vi "Plot Load maker V2.vi"(8 "error in (no error)":errorcluster, 11 "Refs":T6) -> (0 "error out":errorcluster, 3 "Plot config":T1={"plots"=[], "X-axis"={"Name Label.Text"="", "Style"=0, "Tick Colors:Minor Tick Color"=0, "Tick Colors:Tick Color"=0, "Marker Colors:Text Color"=0, "Grid Colors:Major Color"=0, "Grid Colors:Minor Color"=0, "Mapping Mode"=0, "Flipped"=FALSE, "Name Label.Visible"=FALSE, "Name Label.Text Colors:Text Color"=0, "Scale Fit"=0, "Range:Maximum"=0.0, "Range:Minimum"=0.0, "Offset and Multiplier:Multiplier"=0.0, "Offset and Multiplier:Offset"=0.0, "Name Label.Font:Size"=0, "Marker.Font:Size"=0, "Uniform Marker Spacing?"=TRUE, "Format String"=""}, "Y-axes"=[], "General"={"Title"="", "Time to Plot"=1800.0, "Title.Visible"=FALSE, "Sidebar.Visible"=FALSE, "Plot Area:Colors:BG Color"=0, "X Scale.Plot Name"="", "X Scale.Use Plot Name"=FALSE}} {"General"."Time to Plot" format="%<%M:%S>t"})   [LabVIEW 2021, in "RocketPlot.lvlib"]
uses:
  RocketPlot.lvlib
  TypeDefs/Plot UI references.ctl
  Classes/RocketPlotHandle/RocketPlotHandle.lvclass
  <userlib>/bjustice/TipStripOOPanel/Classes/TipPanelHandle/TipPanelHandle.lvclass
  TypeDefs/Plot top row.ctl
  TypeDefs/plot load data V2.ctl
  TypeDefs/plot properties V2.ctl
  TypeDefs/plot attributes V2.ctl
  TypeDefs/Plot scale axis properties.ctl
  TypeDefs/Plot general properties.ctl
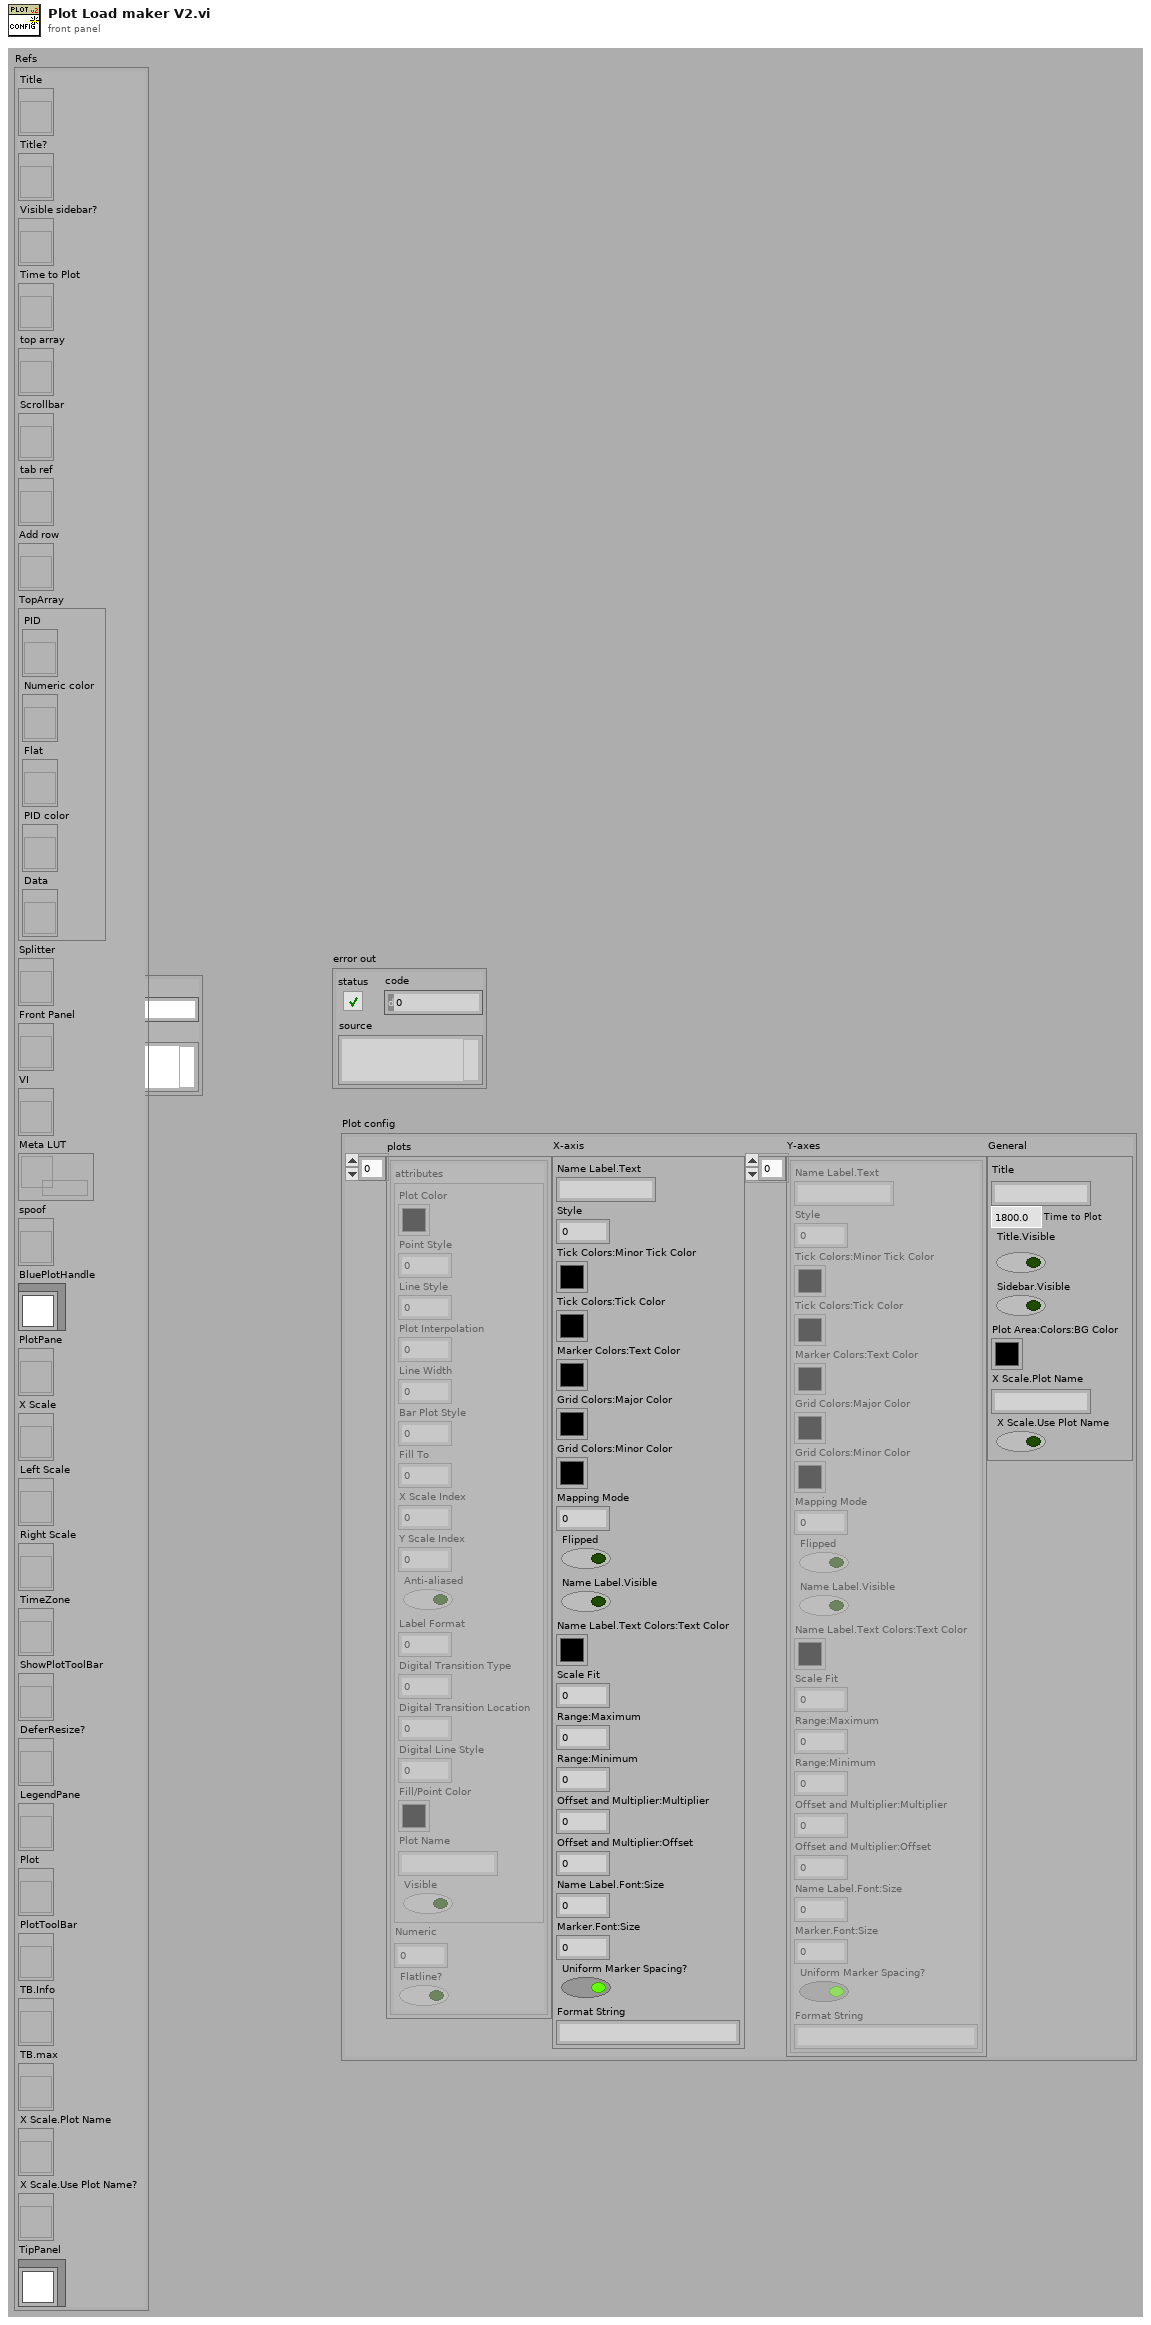
[diagram p1: front panel]
types:
  T1 = typedef "RocketPlot.lvlib/plot load data V2.ctl" = cluster{"plots":T2[], "X-axis":T4, "Y-axes":T4[], "General":T5}
  T2 = typedef "RocketPlot.lvlib/plot properties V2.ctl" = cluster{"attributes":T3, "Numeric":dbl, "Flatline?":bool}
  T3 = typedef "RocketPlot.lvlib/plot attributes V2.ctl" = cluster{"Plot Color":u32, "Point Style":u8, "Line Style":u8, "Plot Interpolation":u8, "Line Width":u8, "Bar Plot Style":u8, "Fill To":i16, "X Scale Index":u32, "Y Scale Index":u32, "Anti-aliased":bool, "Label Format":u8, "Digital Transition Type":u8, "Digital Transition Location":u8, "Digital Line Style":u8, "Fill/Point Color":u32, "Plot Name":string, "Visible":bool}
  T4 = typedef "RocketPlot.lvlib/Plot scale axis properties.ctl" = cluster{"Name Label.Text":string, "Style":u8, "Tick Colors:Minor Tick Color":u32, "Tick Colors:Tick Color":u32, "Marker Colors:Text Color":u32, "Grid Colors:Major Color":u32, "Grid Colors:Minor Color":u32, "Mapping Mode":u8, "Flipped":bool, "Name Label.Visible":bool, "Name Label.Text Colors:Text Color":u32, "Scale Fit":u8, "Range:Maximum":dbl, "Range:Minimum":dbl, "Offset and Multiplier:Multiplier":dbl, "Offset and Multiplier:Offset":dbl, "Name Label.Font:Size":u32, "Marker.Font:Size":u32, "Uniform Marker Spacing?":bool, "Format String":string}
  T5 = typedef "RocketPlot.lvlib/Plot general properties.ctl" = cluster{"Title":string, "Time to Plot":dbl, "Title.Visible":bool, "Sidebar.Visible":bool, "Plot Area:Colors:BG Color":u32, "X Scale.Plot Name":string, "X Scale.Use Plot Name":bool}
  T6 = typedef "RocketPlot.lvlib/Plot UI references.ctl" = cluster{"Title":refnum<vi>, "Title?":refnum<vi>, "Visible sidebar?":refnum<vi>, "Time to Plot":refnum<vi>, "top array":refnum<vi>, "Scrollbar":refnum<vi>, "tab ref":refnum<vi>, "Add row":refnum<vi>, "TopArray":cluster{"PID":refnum<vi>, "Numeric color":refnum<vi>, "Flat":refnum<vi>, "PID color":refnum<vi>, "Data":refnum<vi>}, "Splitter":refnum<vi>, "Front Panel":refnum<vi>, "VI":refnum<vi>, "Meta LUT":refnum<data-value>, "spoof":refnum<vi>, "BluePlotHandle":refnum<class "RocketPlotHandle.lvclass">, "PlotPane":refnum<vi>, "X Scale":refnum<vi>, "Left Scale":refnum<vi>, "Right Scale":refnum<vi>, "TimeZone":refnum<vi>, "ShowPlotToolBar":refnum<vi>, "DeferResize?":refnum<vi>, "LegendPane":refnum<vi>, "Plot":refnum<vi>, "PlotToolBar":refnum<vi>, "TB.Info":refnum<vi>, "TB.max":refnum<vi>, "X Scale.Plot Name":refnum<vi>, "X Scale.Use Plot Name?":refnum<vi>, "TipPanel":refnum<class "TipPanelHandle.lvclass">}
  T7 = typedef "Plot top row.ctl" = cluster{"PID":string, "index":i32, "PID color":u32, "right axis?":bool, "Flatline?":bool, "Numeric color":u32, "Data":string, "Flat":string}
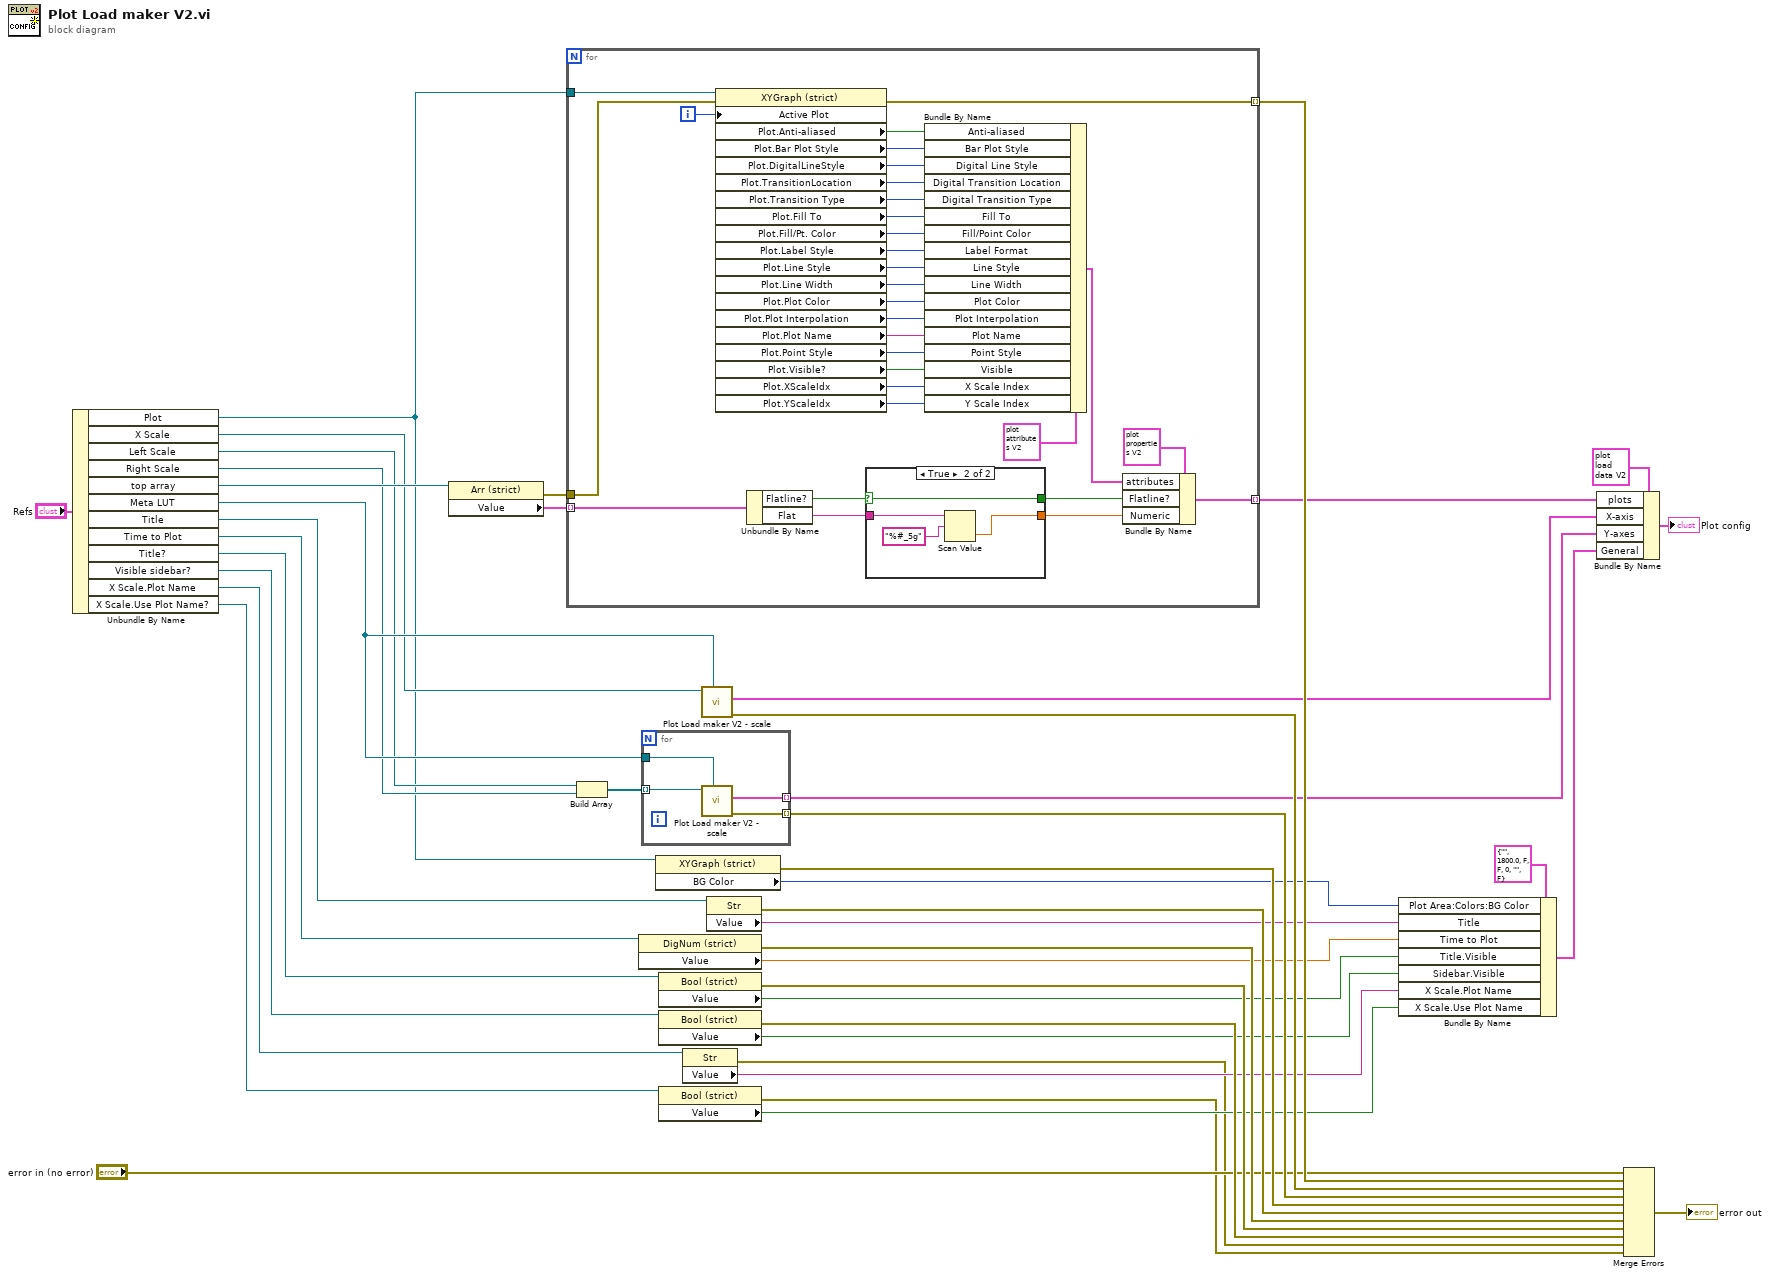
[diagram p0: block diagram]
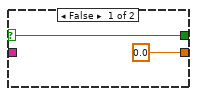
[diagram p2: hidden frame]
diagram:
  n1 = Unbundle By Name("Refs") -> ("Plot"=w7:refnum<vi>, "X Scale"=w11:refnum<vi>, "Left Scale"=w10:refnum<vi>, "Right Scale"=w9:refnum<vi>, "top array"=w32:refnum<vi>, "Meta LUT"=w12:refnum<data-value>, "Title"=w26:refnum<vi>, "Time to Plot"=w25:refnum<vi>, "Title?"=w24:refnum<vi>, "Visible sidebar?"=w23:refnum<vi>, "X Scale.Plot Name"=w6:refnum<vi>, "X Scale.Use Plot Name?"=w5:refnum<vi>)
  n2 = property class="Arr (strict)"(reference=w32) -> (error out=w17:errorcluster, "Value"=w31:T7[])  [unwired: 1 in, 1 out]
  n3 = for {
    tunnel: w7 -> [w54]
    tunnel: w31 -> [w52] mode=indexing
    tunnel: [w45] -> w30 mode=indexing
    tunnel: [w44] -> w41 mode=indexing
    tunnel: w17 -> [w43]
    i -> [w53]
    n4 = property class="XYGraph (strict)"(reference=w54, error in=w43, "Active Plot"=w53) -> (error out=w44:errorcluster, "Plot.Anti-aliased"=w71:bool, "Plot.Bar Plot Style"=w70:u8, "Plot.DigitalLineStyle"=w69:u8, "Plot.TransitionLocation"=w68:u8, "Plot.Transition Type"=w67:u8, "Plot.Fill To"=w66:i16, "Plot.Fill/Pt. Color"=w65:u32, "Plot.Label Style"=w64:u8, "Plot.Line Style"=w63:u8, "Plot.Line Width"=w62:u8, "Plot.Plot Color"=w61:u32, "Plot.Plot Interpolation"=w60:u8, "Plot.Plot Name"=w59:string, "Plot.Point Style"=w58:u8, "Plot.Visible?"=w57:bool, "Plot.XScaleIdx"=w56:u32, "Plot.YScaleIdx"=w55:u32)  [unwired: 1 out]
    n5 = Unbundle By Name(w52) -> ("Flatline?"=w49:bool, "Flat"=w48:string)
    n6 = case shown="True" w49 {
      selector: w49 -> [w74 w78]
      tunnel: w48 -> [_ w77]
      tunnel: [w74 w78] -> w47
      tunnel: [0.0 ("Numeric") w75] -> w46
      frame False {
      }
      frame True {
        n7 = Scan Value(string=w77, format string="%#_5g") -> (value=w75:dbl)  [unwired: 1 in, 1 out]
      }
    }
    n8 = Bundle By Name(cluster=T3 {"Plot Color"=0, "Point Style"=0, "Line Style"=0, "Plot Interpolation"=0, "Line Width"=0, "Bar Plot Style"=0, "Fill To"=0, "X Scale Index"=0, "Y Scale Index"=0, "Anti-aliased"=FALSE, "Label Format"=0, "Digital Transition Type"=0, "Digital Transition Location"=0, "Digital Line Style"=0, "Fill/Point Color"=0, "Plot Name"="", "Visible"=FALSE} ("attributes"), "Anti-aliased"=w71, "Bar Plot Style"=w70, "Digital Line Style"=w69, "Digital Transition Location"=w68, "Digital Transition Type"=w67, "Fill To"=w66, "Fill/Point Color"=w65, "Label Format"=w64, "Line Style"=w63, "Line Width"=w62, "Plot Color"=w61, "Plot Interpolation"=w60, "Plot Name"=w59, "Point Style"=w58, "Visible"=w57, "X Scale Index"=w56, "Y Scale Index"=w55) -> (w50:T3)
    n9 = Bundle By Name(cluster=T2 {"attributes"={"Plot Color"=0, "Point Style"=0, "Line Style"=0, "Plot Interpolation"=0, "Line Width"=0, "Bar Plot Style"=0, "Fill To"=0, "X Scale Index"=0, "Y Scale Index"=0, "Anti-aliased"=FALSE, "Label Format"=0, "Digital Transition Type"=0, "Digital Transition Location"=0, "Digital Line Style"=0, "Fill/Point Color"=0, "Plot Name"="", "Visible"=FALSE}, "Numeric"=0.0, "Flatline?"=FALSE} ("Cluster"), "attributes"=w50, "Flatline?"=w47, "Numeric"=w46) -> (w45:T2)
  }
  n10 = Build Array(w10, w9) -> (w8:refnum<vi>[])
  n11 = property class="DigNum (strict)"(reference=w25) -> (error out=w37:errorcluster, "Value"=w21:dbl)  [unwired: 1 in, 1 out]
  n12 = for {
    tunnel: [w82] -> w28 mode=indexing
    tunnel: [w81] -> w39 mode=indexing
    tunnel: w12 -> [w80]
    tunnel: w8 -> [w79] mode=indexing
    n13 = call "Plot Load maker V2 - scale.vi"("Meta LUT"=w80, "Scale reference"=w79) -> ("error out"=w81:errorcluster, "Axis config"=w82:T4)  [unwired: 7 in, 1 out]
  }
  n14 = property class="XYGraph (strict)"(reference=w7) -> (error out=w42:errorcluster, "BG Color"=w13:u32)  [unwired: 1 in, 1 out]
  n15 = property class="Bool (strict)"(reference=w24) -> (error out=w36:errorcluster, "Value"=w20:bool)  [unwired: 1 in, 1 out]
  n16 = property class="Bool (strict)"(reference=w23) -> (error out=w35:errorcluster, "Value"=w19:bool)  [unwired: 1 in, 1 out]
  n17 = property class="Bool (strict)"(reference=w5) -> (error out=w1:errorcluster, "Value"=w3:bool)  [unwired: 1 in, 1 out]
  n18 = property class="Str"(reference=w6) -> (error out=w2:errorcluster, "Value"=w4:string)  [unwired: 1 in, 1 out]
  n19 = call "Plot Load maker V2 - scale.vi"("Meta LUT"=w12, "Scale reference"=w11) -> ("error out"=w40:errorcluster, "Axis config"=w29:T4)  [unwired: 7 in, 1 out]
  n20 = property class="Str"(reference=w26) -> (error out=w38:errorcluster, "Value"=w22:string)  [unwired: 1 in, 1 out]
  n21 = Bundle By Name(cluster=T5 {"Title"="", "Time to Plot"=1800.0, "Title.Visible"=FALSE, "Sidebar.Visible"=FALSE, "Plot Area:Colors:BG Color"=0, "X Scale.Plot Name"="", "X Scale.Use Plot Name"=FALSE} ("General"), "Plot Area:Colors:BG Color"=w13, "Title"=w22, "Time to Plot"=w21, "Title.Visible"=w20, "Sidebar.Visible"=w19, "X Scale.Plot Name"=w4, "X Scale.Use Plot Name"=w3) -> (w18:T5)
  n22 = Bundle By Name(cluster=T1 {"plots"=[], "X-axis"={"Name Label.Text"="", "Style"=0, "Tick Colors:Minor Tick Color"=0, "Tick Colors:Tick Color"=0, "Marker Colors:Text Color"=0, "Grid Colors:Major Color"=0, "Grid Colors:Minor Color"=0, "Mapping Mode"=0, "Flipped"=FALSE, "Name Label.Visible"=FALSE, "Name Label.Text Colors:Text Color"=0, "Scale Fit"=0, "Range:Maximum"=0.0, "Range:Minimum"=0.0, "Offset and Multiplier:Multiplier"=0.0, "Offset and Multiplier:Offset"=0.0, "Name Label.Font:Size"=0, "Marker.Font:Size"=0, "Uniform Marker Spacing?"=TRUE, "Format String"=""}, "Y-axes"=[], "General"={"Title"="", "Time to Plot"=1800.0, "Title.Visible"=FALSE, "Sidebar.Visible"=FALSE, "Plot Area:Colors:BG Color"=0, "X Scale.Plot Name"="", "X Scale.Use Plot Name"=FALSE}} ("Cluster"), "plots"=w30, "X-axis"=w29, "Y-axes"=w28, "General"=w18) -> (→"Plot config":T1)
  n23 = Merge Errors("error in (no error)", w41, w40, w39, w42, w38, w37, w36, w35, w2, w1) -> (→"error out":errorcluster)
